vi "Receiver.vi"() -> ()   [LabVIEW 2020]
uses:
  <vilib>/httpClient/LabVIEWHTTPClient.lvlib
panel:
  out "value":cluster{"Message":string}
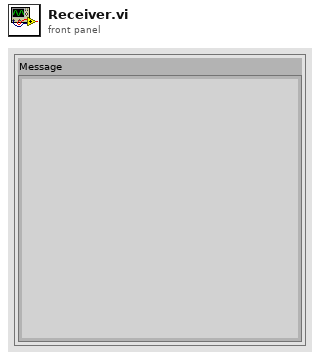
[diagram p1: front panel]
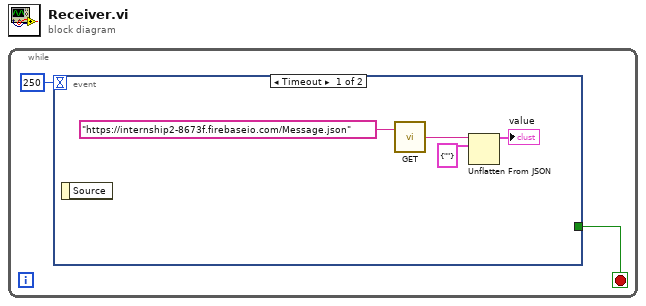
[diagram p0: block diagram]
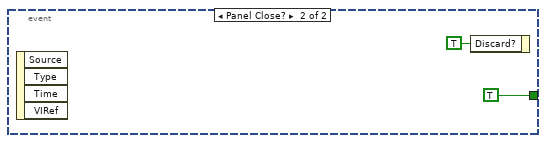
[diagram p2: hidden frame]
diagram:
  n1 = while {
    stop <- w1 stop-if-true
    n2 = event shown="[0] Timeout" {
      selector: _ -> [_ _]
      dyn-events: _ -> [_ _]
      timeout: 250 -> [_ _]
      tunnel: [_ TRUE] -> w1
      event Timeout {
        n3 = event-data() -> ()  [unwired: 1 in, 1 out]
        n4 = call <vilib>:"GET.vi"("url"="https://internship2-8673f.firebaseio.com/Message.json") -> ("body"=w4:string)  [unwired: 11 in, 3 out]
        n5 = Unflatten From JSON(JSON string=w4, type and defaults=cluster{"Message":string} {"Message"=""} ("Cluster")) -> (value=→"value":cluster{"Message":string})  [unwired: 5 in, 1 out]
      }
      event Panel Close? {
        n6 = event-data() -> ()  [unwired: 1 in, 4 out]
        n7 = event-data("Discard?"=TRUE) -> ()  [unwired: 1 in, 1 out]
      }
    }
  }
